vi "Build HTTP Header.vi"(10 "POST Data Length":i32, 11 "DeepL Free API?":bool) -> (3 "Array":cluster{"header":string, "value":string}[](array[cluster]))   [LabVIEW 2015, in "lv-deepl-api.lvlib"]
uses:
  lv-deepl-api.lvlib
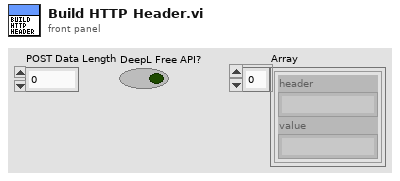
[diagram p1: front panel]
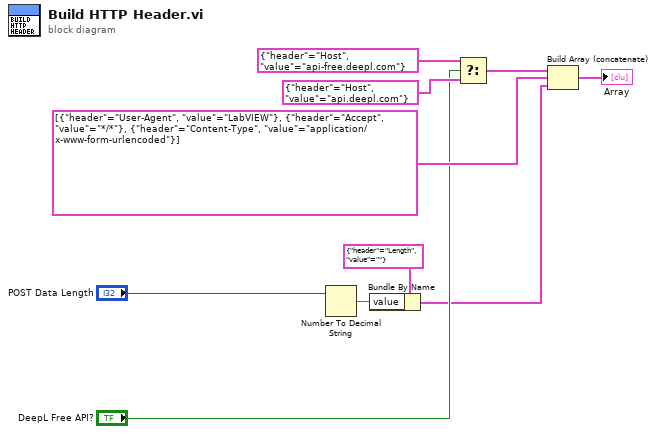
[diagram p0: block diagram]
diagram:
  n1 = Number To Decimal String(number="POST Data Length") -> (decimal integer string=w5:string)  [unwired: 1 in]
  n2 = Bundle By Name(cluster=cluster{"header":string, "value":string} {"header"="Length", "value"=""} ("Cluster"), "value"=w5) -> (w2:cluster{"header":string, "value":string})
  n3 = Select(t=cluster{"header":string, "value":string} {"header"="Host", "value"="api-free.deepl.com"} ("Cluster"), s="DeepL Free API?", f=cluster{"header":string, "value":string} {"header"="Host", "value"="api.deepl.com"} ("Cluster")) -> (s? t:f=w9:cluster{"header":string, "value":string})
  n4 = Build Array (concatenate)(w9, cluster{"header":string, "value":string}[] [{"header"="User-Agent", "value"="LabVIEW"}, {"header"="Accept", "value"="*/*"}, {"header"="Content-Type", "value"="application/x-www-form-urlencoded"}], w2) -> (→"Array":cluster{"header":string, "value":string}[])
